vi "Distinguished by type.vi"() -> ()   [LabVIEW 2012]
uses:
  Madlib.dll
  <vilib>/measure/NI_MABase.lvlib
panel:
  in  "Device Type to control Z":i32
  in  "Device Type to control\nX & Y":i32
  out "Z Position um":dbl(graph)
  in  "Z Offset um":dbl=50.0 min=0.0 max=200.0 step=1.0 format="%.3f"
  in  "Y Offset um":dbl=50.0 min=0.0 max=200.0 step=1.0 format="%.3f"
  out "Y Position um":dbl(graph)
  in  "Signal type":T1(ring)
  in  "Amplitude (um)":dbl=10.0 min=0.0 max=100.0 step=0.1 format="%.3f"
  in  "X Offset um":dbl=50.0 min=0.0 max=200.0 step=1.0 format="%.3f"
  out "X Position um":dbl(graph)
  in  "?":bool
  # "This example VI replicates MonitorXYZ.vi using multiple Nano-Drive's.  One Nano-Drive controls the XY axis and the\nother controls Z.  The Nano-Drives are differentiated by their types."
  # "USB 1.1     USB2.0\nSingle Axis              4096             8193\nSingle Axis(20 bit)                       8705   \nNanoGuage            8192     \nThree Axis              4144            8195 \nTip / Tilt Z (16 bit)                       8275 \nThree Axis(20 bit)  4656            8707   \nTip / Tilt Z (20 bit)   4691            8787"
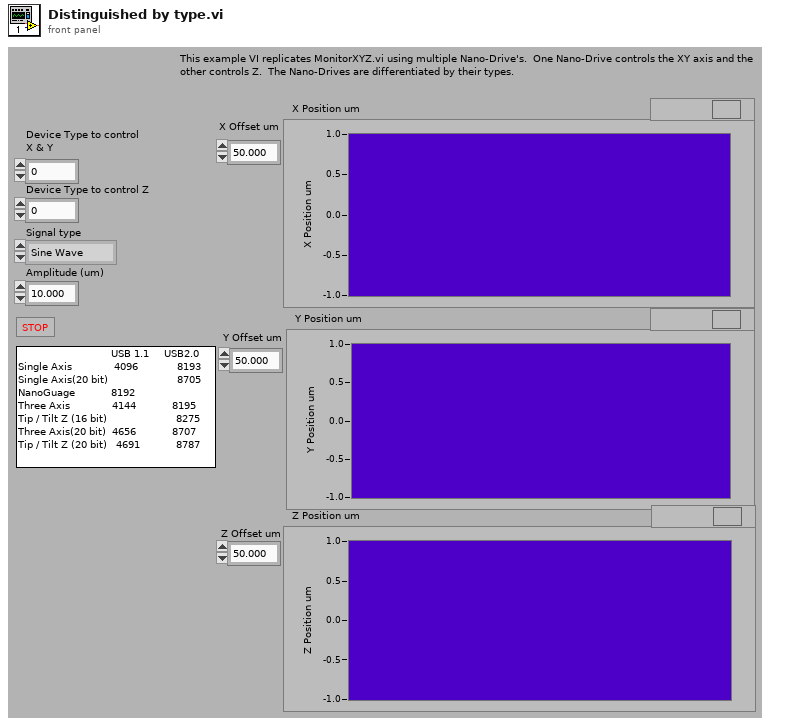
[diagram p1: front panel]
types:
  T1 = enum16{"Sine Wave", "Triangle Wave", "Square Wave", "Sawtooth Wave"}
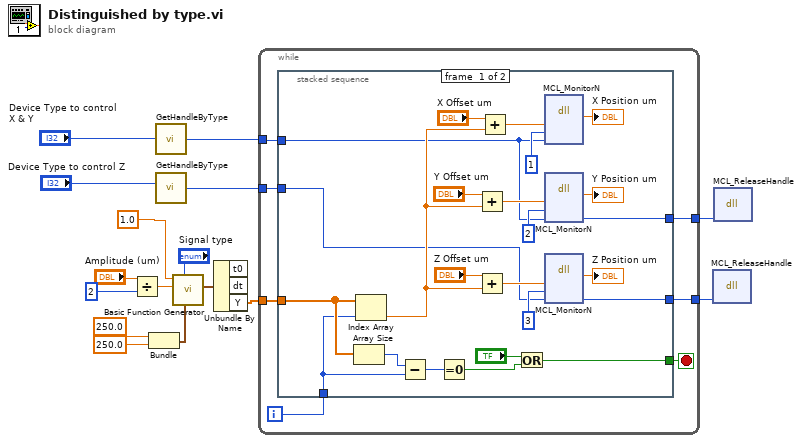
[diagram p0: block diagram]
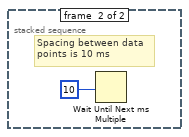
[diagram p2: hidden frame]
diagram:
  n1 = Divide(x="Amplitude (um)", y=2) -> (x/y=w12:dbl)
  n2 = Bundle(250.0, 250.0) -> (w14:cluster{dbl, dbl})  [unwired: 1 in]
  n3 = call "GetHandleByType.vi"("Type"="Device Type to control\nX & Y") -> ("Handle"=w4:i32)
  n4 = call "GetHandleByType.vi"("Type"="Device Type to control Z") -> ("Handle"=w3:i32)
  n5 = call <vilib>:"Basic Function Generator.vi"("sampling info"=w14, "signal type"="Signal type", "amplitude"=w12, "frequency"=1.0) -> ("signal out"=w10:waveform(dbl))  [unwired: 5 in, 2 out]
  n6 = Unbundle By Name ("Get Waveform Components")(w10) -> ("Y"=w8:dbl[])  [unwired: 2 out]
  n7 = while {
    tunnel: w8 -> [w23]
    tunnel: [w19] -> w7
    tunnel: w4 -> [w22]
    tunnel: [w18] -> w5
    tunnel: w3 -> [w17]
    i -> [w21]
    stop <- w20 stop-if-true
    n8 = stacked-sequence {
      tunnel: w23 -> [w44 _]
      tunnel: w22 -> [w24 _]
      tunnel: w21 -> [w29 _]
      tunnel: [w28 _] -> w20
      tunnel: [w27 _] -> w19
      tunnel: [w26 _] -> w18
      tunnel: w17 -> [w25 _]
      frame #0 {
        n9 = Array Size(array=w44) -> (size(s)=w47:i32)
        n10 = Index Array "Index Array"(array=w44, index=w29) -> (element=w36:dbl)
        n11 = Subtract(x=w47, y=w29) -> (x-y=w46:i32)
        n12 = Equal To 0?(x=w46) -> (x = 0?=w45:bool)
        n13 = Add(x="Y Offset um", y=w36) -> (x+y=w41:dbl)
        n14 = Add(x="Z Offset um", y=w36) -> (x+y=w40:dbl)
        n15 = Add(x="X Offset um", y=w36) -> (x+y=w42:dbl)
        n16 = Or(x="?", y=w45) -> (x .or. y?=w28:bool)
        n17 = dll-call lib="C:/Users/Labview/Desktop/SRR/Madlib_x64/Labview Examples/MADLib.dll" fn="MCL_MonitorN"("position"=w42, "axis"=u16 1, "handle"=w24) -> (→"X Position um":dbl)  [unwired: 6 in, 2 out]
        n18 = dll-call lib="C:/Users/Labview/Desktop/SRR/Madlib_x64/Labview Examples/MADLib.dll" fn="MCL_MonitorN"("position"=w41, "axis"=u16 2, "handle"=w24) -> (→"Y Position um":dbl, "handle"=w27:i32)  [unwired: 5 in, 2 out]
        n19 = dll-call lib="C:/Users/Labview/Desktop/SRR/Madlib_x64/Labview Examples/MADLib.dll" fn="MCL_MonitorN"("position"=w40, "axis"=3, "handle"=w25) -> (→"Z Position um":dbl, "handle"=w26:i32)  [unwired: 5 in, 2 out]
      }
      frame #1 {
        # "Spacing between data\npoints is 10 ms"
        n20 = Wait Until Next ms Multiple(millisecond multiple=10) -> ()  [unwired: 1 out]
      }
    }
  }
  n21 = dll-call lib="C:/Users/Labview/Desktop/SRR/Madlib_x64/Labview Examples/MADLib.dll" fn="MCL_ReleaseHandle"("handle"=w5) -> ()  [unwired: 5 in, 2 out]
  n22 = dll-call lib="C:/Users/Labview/Desktop/SRR/Madlib_x64/Labview Examples/MADLib.dll" fn="MCL_ReleaseHandle"("handle"=w7) -> ()  [unwired: 5 in, 2 out]
